vi "Refnum to DVR.vi"(11 "Refnum out":T1) -> (3 "Data Value Reference in":refnum<data-value>)   [LabVIEW 2019, in "HTTP Client Extensions.lvlib" / "Get Async.lvlib"]
uses:
  Get Async.lvlib
  HTTP GET Async/GET Async.lvclass
  controls/Refnum Type - Enum.ctl
  controls/Refnum Type.ctl
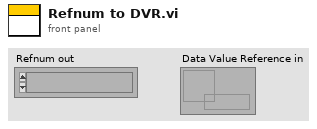
[diagram p1: front panel]
types:
  T1 = typedef "HTTP Client Extensions.lvlib/Get Async.lvlib/Refnum Type.ctl" = refnum<k1>
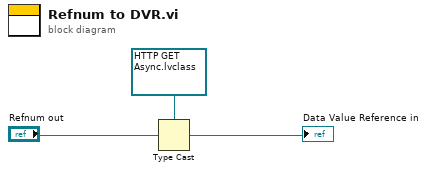
[diagram p0: block diagram]
diagram:
  n1 = Type Cast(type=refnum<data-value> refnum ("Data Value Reference in"), x="Refnum out") -> (*(type *) &x=→"Data Value Reference in":refnum<data-value>)
